vi "PCO_ball_puff_pupil_FLIR_trig_2024_JMR.vi"() -> ()   [LabVIEW 2020]
uses:
  C:/Users/jqr5792/AppData/Roaming/PCO Digital Camera Toolbox/pco.labview/pco.camera/Controls/binning.ctl
  <vilib>/vision/driver/IMAQdx.llb/IMAQdx Camera Control Mode.ctl
  <vilib>/userDefined/High Color/IMAQdx.ctl
  <vilib>/vision/driver/IMAQdx.llb/IMAQdx Acquisition Mode.ctl
  C:/Users/jqr5792/AppData/Roaming/PCO Digital Camera Toolbox/pco.labview/pco.camera/Camera.lvclass
  <vilib>/vision/driver/IMAQdx.llb/IMAQdx Buffer Number Mode.ctl
  7076c1c6-cf5a-4733-8e55-1dfd44238ec2.vi
  <vilib>/DAQmx/write.llb/DAQmx Write (Digital Bool 1Line 1Point).vi
  <vilib>/DAQmx/read.llb/DAQmx Read (Analog 1D Wfm NChan NSamp).vi
  <vilib>/DAQmx/write.llb/DAQmx Write (Digital 1D Bool NChan 1Samp 1Line).vi
  <vilib>/DAQmx/create/channels.llb/DAQmx Create Channel (AI-Voltage-Basic).vi
  <vilib>/DAQmx/configure/timing.llb/DAQmx Timing (Sample Clock).vi
  <vilib>/DAQmx/configure/trigger.llb/DAQmx Start Trigger (Digital Edge).vi
  <vilib>/DAQmx/create/channels.llb/DAQmx Create Channel (DO-Digital Output).vi
  <vilib>/DAQmx/create/channels.llb/DAQmx Create Channel (CO-Pulse Generation-Frequency).vi
  <vilib>/DAQmx/configure/timing.llb/DAQmx Timing (Implicit).vi
  <vilib>/DAQmx/miscellaneous.llb/DAQmx Fill In Error Info.vi
  <vilib>/vision/driver/NI_Vision_Acquisition_Software.lvlib
panel:
  out "New Lost":u32
  out "NewNumLost":u32[](array[numeric])
  out "NewBuffNum":u32[](array[numeric])
  out "Buffer Number Out":u32
  out "Min/Sec for trial":cluster{dbl, dbl}
  in  "No stim":dbl=1.0
  out "n total images":i32
  out "PCO Frame Rate":dbl
  out "Time Elapsed (s)":u32
  out "Recorded Images":u32=7194
  out "PCO Recording":bool=TRUE
  in  "ROI":cluster{"x0":u64, "y0":u64, "x1":u64, "y1":u64}={"x0"=100, "y0"=175, "x1"=500, "y1"=425}
  in  "Binning":T1={"vert"=4, "horz"=4}
  in  "TriggerMode":T2(ring)=enum."external exposure start"
  in  "Exposure [s]":dbl=0.008 min=0.0005 max=2.0 step=0.001
  out "Image":T3(plugin-control)
  out "Last Whisk\nBuffer":u32=488
  out "Actual WhiskCam\nFrame Rate":dbl(knob)=148.05583250249254 scale=0.0..300.0
  out "Pupil":T3(plugin-control)
  out "Solenoids":bool[](array[boolean])
  in  "Stim \nOffset (s)":dbl=15.0
  in  "Puff \nDuration (s)":dbl=0.1 step=0.1
  in  "Inter-Stim\nInterval (s)":dbl=30.0
  in  "Stim only":dbl=5.0
  in  "Auditory control":dbl=2.0
  in  "Left Pad":tag="Dev1/port0/line1"
  in  "Right Pad":tag="Dev1/port0/line3"
  in  "Squeeze":tag="Dev1/port0/line2"
  out "Analog Data":bool
  out "Analog acquisition length":i32
  in  "Channel Labels":string[](array[string])=["BallVelocity", "LeftPad", "Control", "RightPad", "Broadband", "LFP", "MUA"]
  in  "physical channels":tag="Dev1/ai0:6"
  in  "Analog Acquisition Setup":cluster{"Analog Sampling Rate":u16}={"Analog Sampling Rate"=5000} {"Analog Sampling Rate" format="%0.0f"}
  in  "Camera Acquisition Setup":cluster{"CBVCam Rate":u16, "WebCam Rate":u16}={"CBVCam Rate"=60, "WebCam Rate"=30}
  out "Notes Size":i32=7
  out "Notes Reversed":string[](array[string])=["Experimenter", "Animal ID", "Imaged Hemisphere", "Solenoid Pressure", "Isoflurane time", "Session ID", "Amplifier Gain"]
  out "Notes Array":string[](array[string])=["Amplifier Gain", "Session ID", "Isoflurane time", "Solenoid Pressure", "Imaged Hemisphere", "Animal ID", "Experimenter"]
  in  "Session Notes:":T4={"Experimenter"="Joe Ricotta", "Animal ID"="T31", "Imaged Hemisphere"="RH", "Solenoid Pressure"="10", "Infusion Compound"="na", "Infusion volume nL"="na", "Infusion rate nlpS"="na", "Block"="1000", "Molar conc um"="na"}
  in  "Target Path":path=path "D:/Joe/sample/PCO_setup" caption="Final saved file location"
  out "Current file name":string="170828_12_37_58"
  out "Actual WebCam Frame Rate":dbl(knob) scale=0.0..30.0
  out "WebCam":T3(plugin-control)
  out "CBV Camera":bool=TRUE
  out "Trial Time Elapsed (Min)":cluster{dbl, dbl}(slide)={0.5, 0.05364406000000001} scale=0.0..17.0
  in  "Temp Path":path=path "C:/LabView Direct Files" caption="Temporary path for\nstreamed data"
  in  "Stop":bool
  # "File Settings:"
  # "Binning: 4,4"
  # "roi: 50, 200, 600, 400"
  # "Left Pad"
  # "Control"
  # "Right"
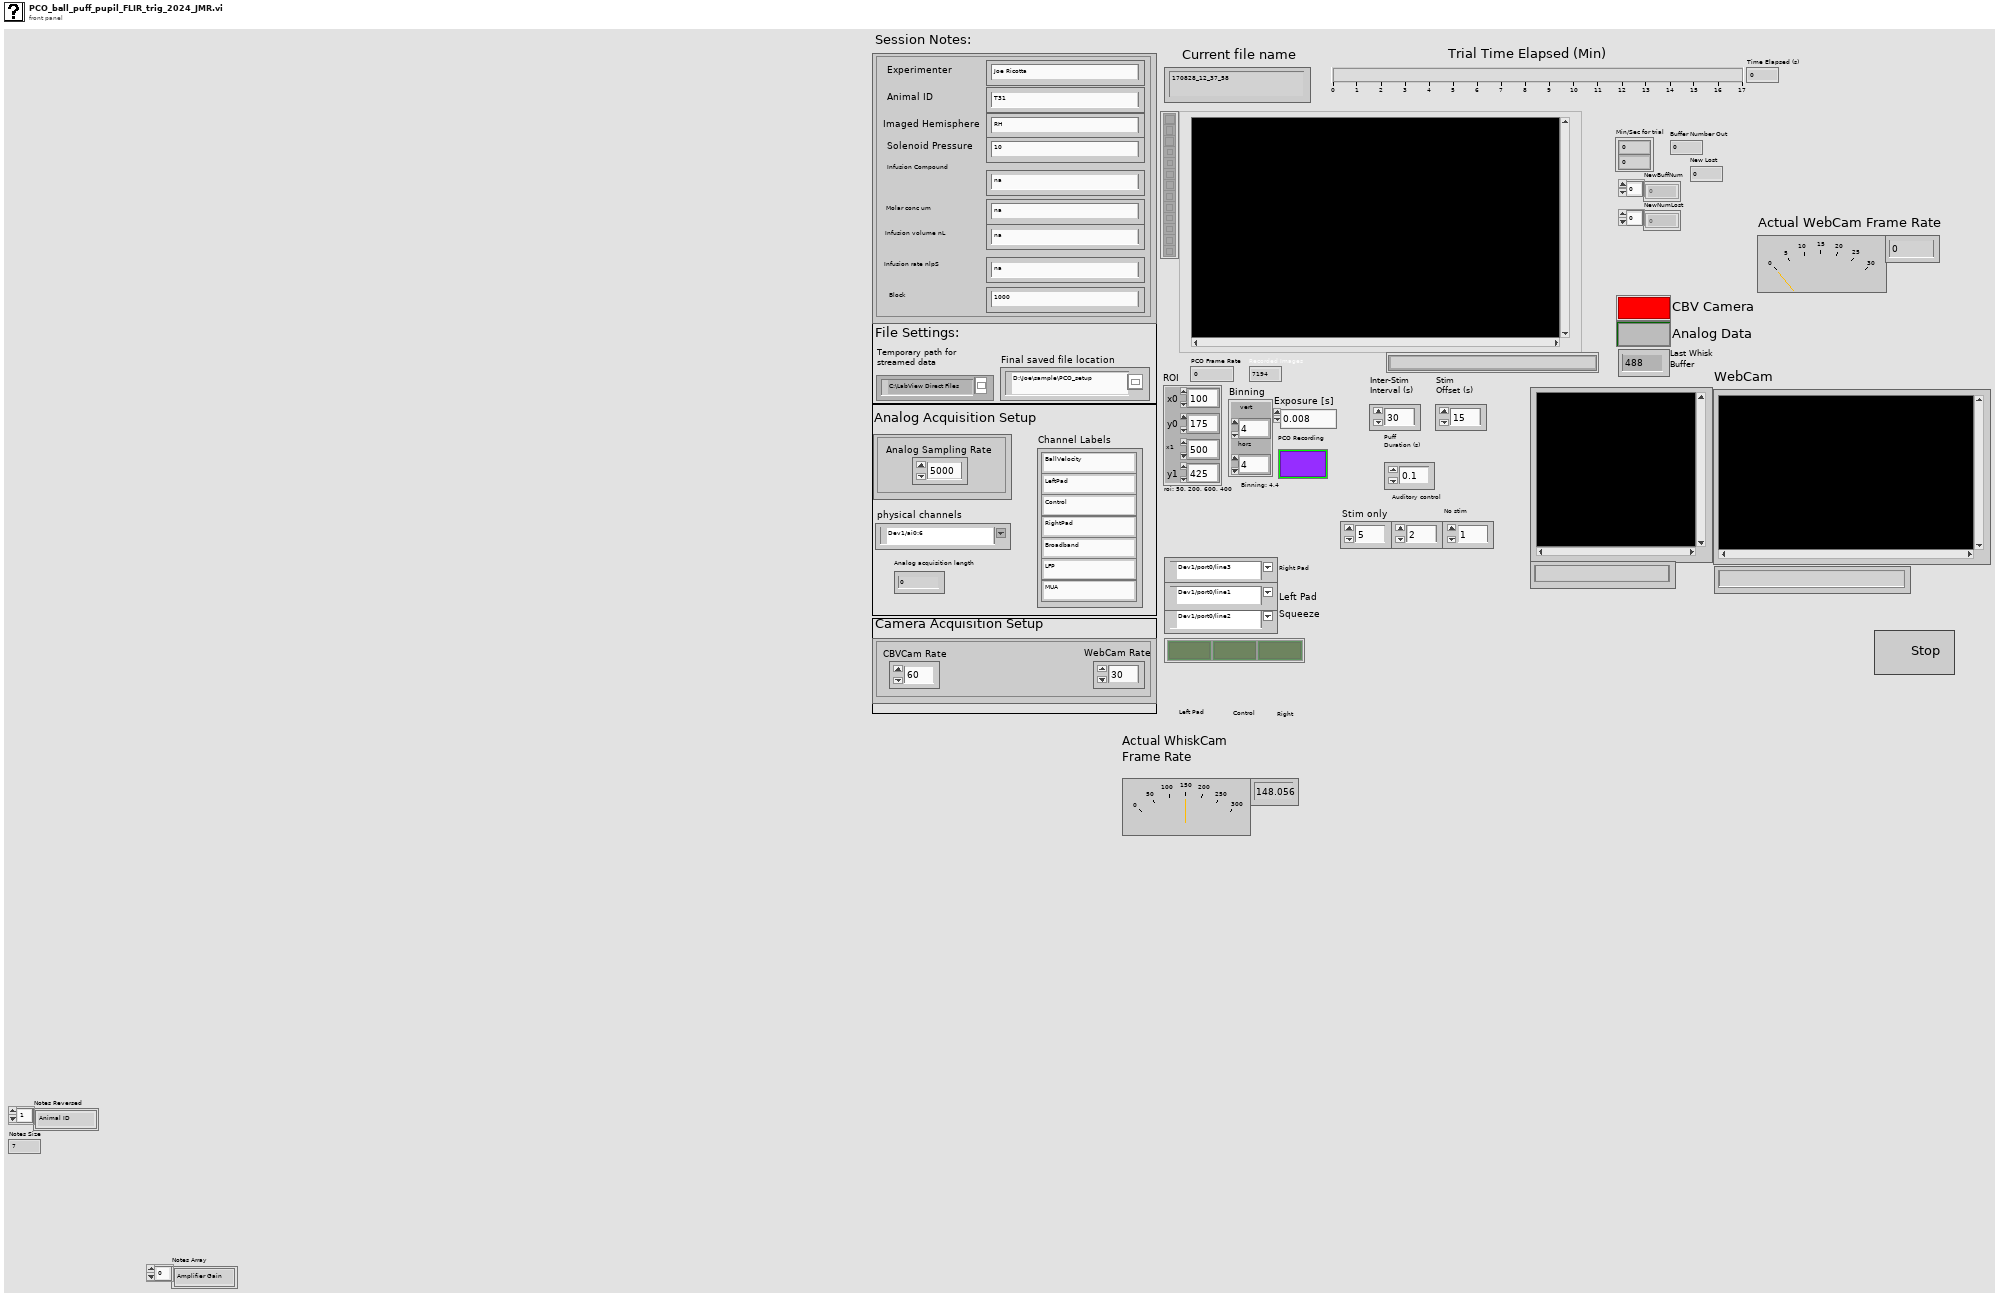
[diagram p1: front panel]
types:
  T1 = typedef "Camera.lvclass/binning.ctl" = cluster{"vert":u16, "horz":u16}
  T2 = enum16{"auto sequence", "software trigger", "external exposure start", "external exposure control"}
  T3 = typedef "IMAQ Image.ctl" = refnum<image>
  T4 = cluster{"Experimenter":string, "Animal ID":string, "Imaged Hemisphere":string, "Solenoid Pressure":string, "Infusion Compound":string, "Infusion volume nL":string, "Infusion rate nlpS":string, "Block":string, "Molar conc um":string}
  T5 = typedef "IMAQdx.ctl" = refnum<k21>
  T6 = typedef "Image Type" = u32
  T7 = enum16{"open", "replace", "create", "open or create", "replace or create", "replace or create with confirmation"}
  T8 = typedef "NI_Vision_Acquisition_Software.lvlib/IMAQdx Acquisition Mode.ctl" = enum32{"One Shot", "Continuous"}
  T9 = typedef "NI_Vision_Acquisition_Software.lvlib/IMAQdx Camera Control Mode.ctl" = enum32{"Controller", "Listener"}
  T10 = enum16{"open", "open or create", "create or replace", "create", "open (read-only)"}
  T11 = cluster{"exposure_time_s":dbl, "delay_time_s":dbl, "roi":cluster{"x0":u64, "y0":u64, "x1":u64, "y1":u64}, "timestamp_mode":u16, "pixelrate":u32, "trigger_mode":u16, "acquire_mode":u16, "metadata_mode":u16, "noisefilter_mode":u16, "binning":T1}
  T12 = typedef "IMAQ AVI2 Refnum.ctl" = refnum<k20>
  T13 = enum16{"sequence", "sequence non blocking", "ring buffer", "fifo", "sequence_dpcore", "sequence_non_blocking_dpcore", "ring_buffer_dpcore", "fifo_dpcore", "tif", "multitif", "pcoraw", "b16", "dicom", "multidicom"}
  T14 = enum16{"Undefined", "Mono8", "Mono16", "BGRA8", "RGBA8", "BGRA16", "RGBA16", "CompressedMono8"}
  T15 = enum16{"big-endian, network order", "native, host order", "little-endian"}
  T16 = typedef "NI_Vision_Acquisition_Software.lvlib/IMAQdx Buffer Number Mode.ctl" = enum32{"Next", "Last", "Buffer Number", "Every", "Last New"}
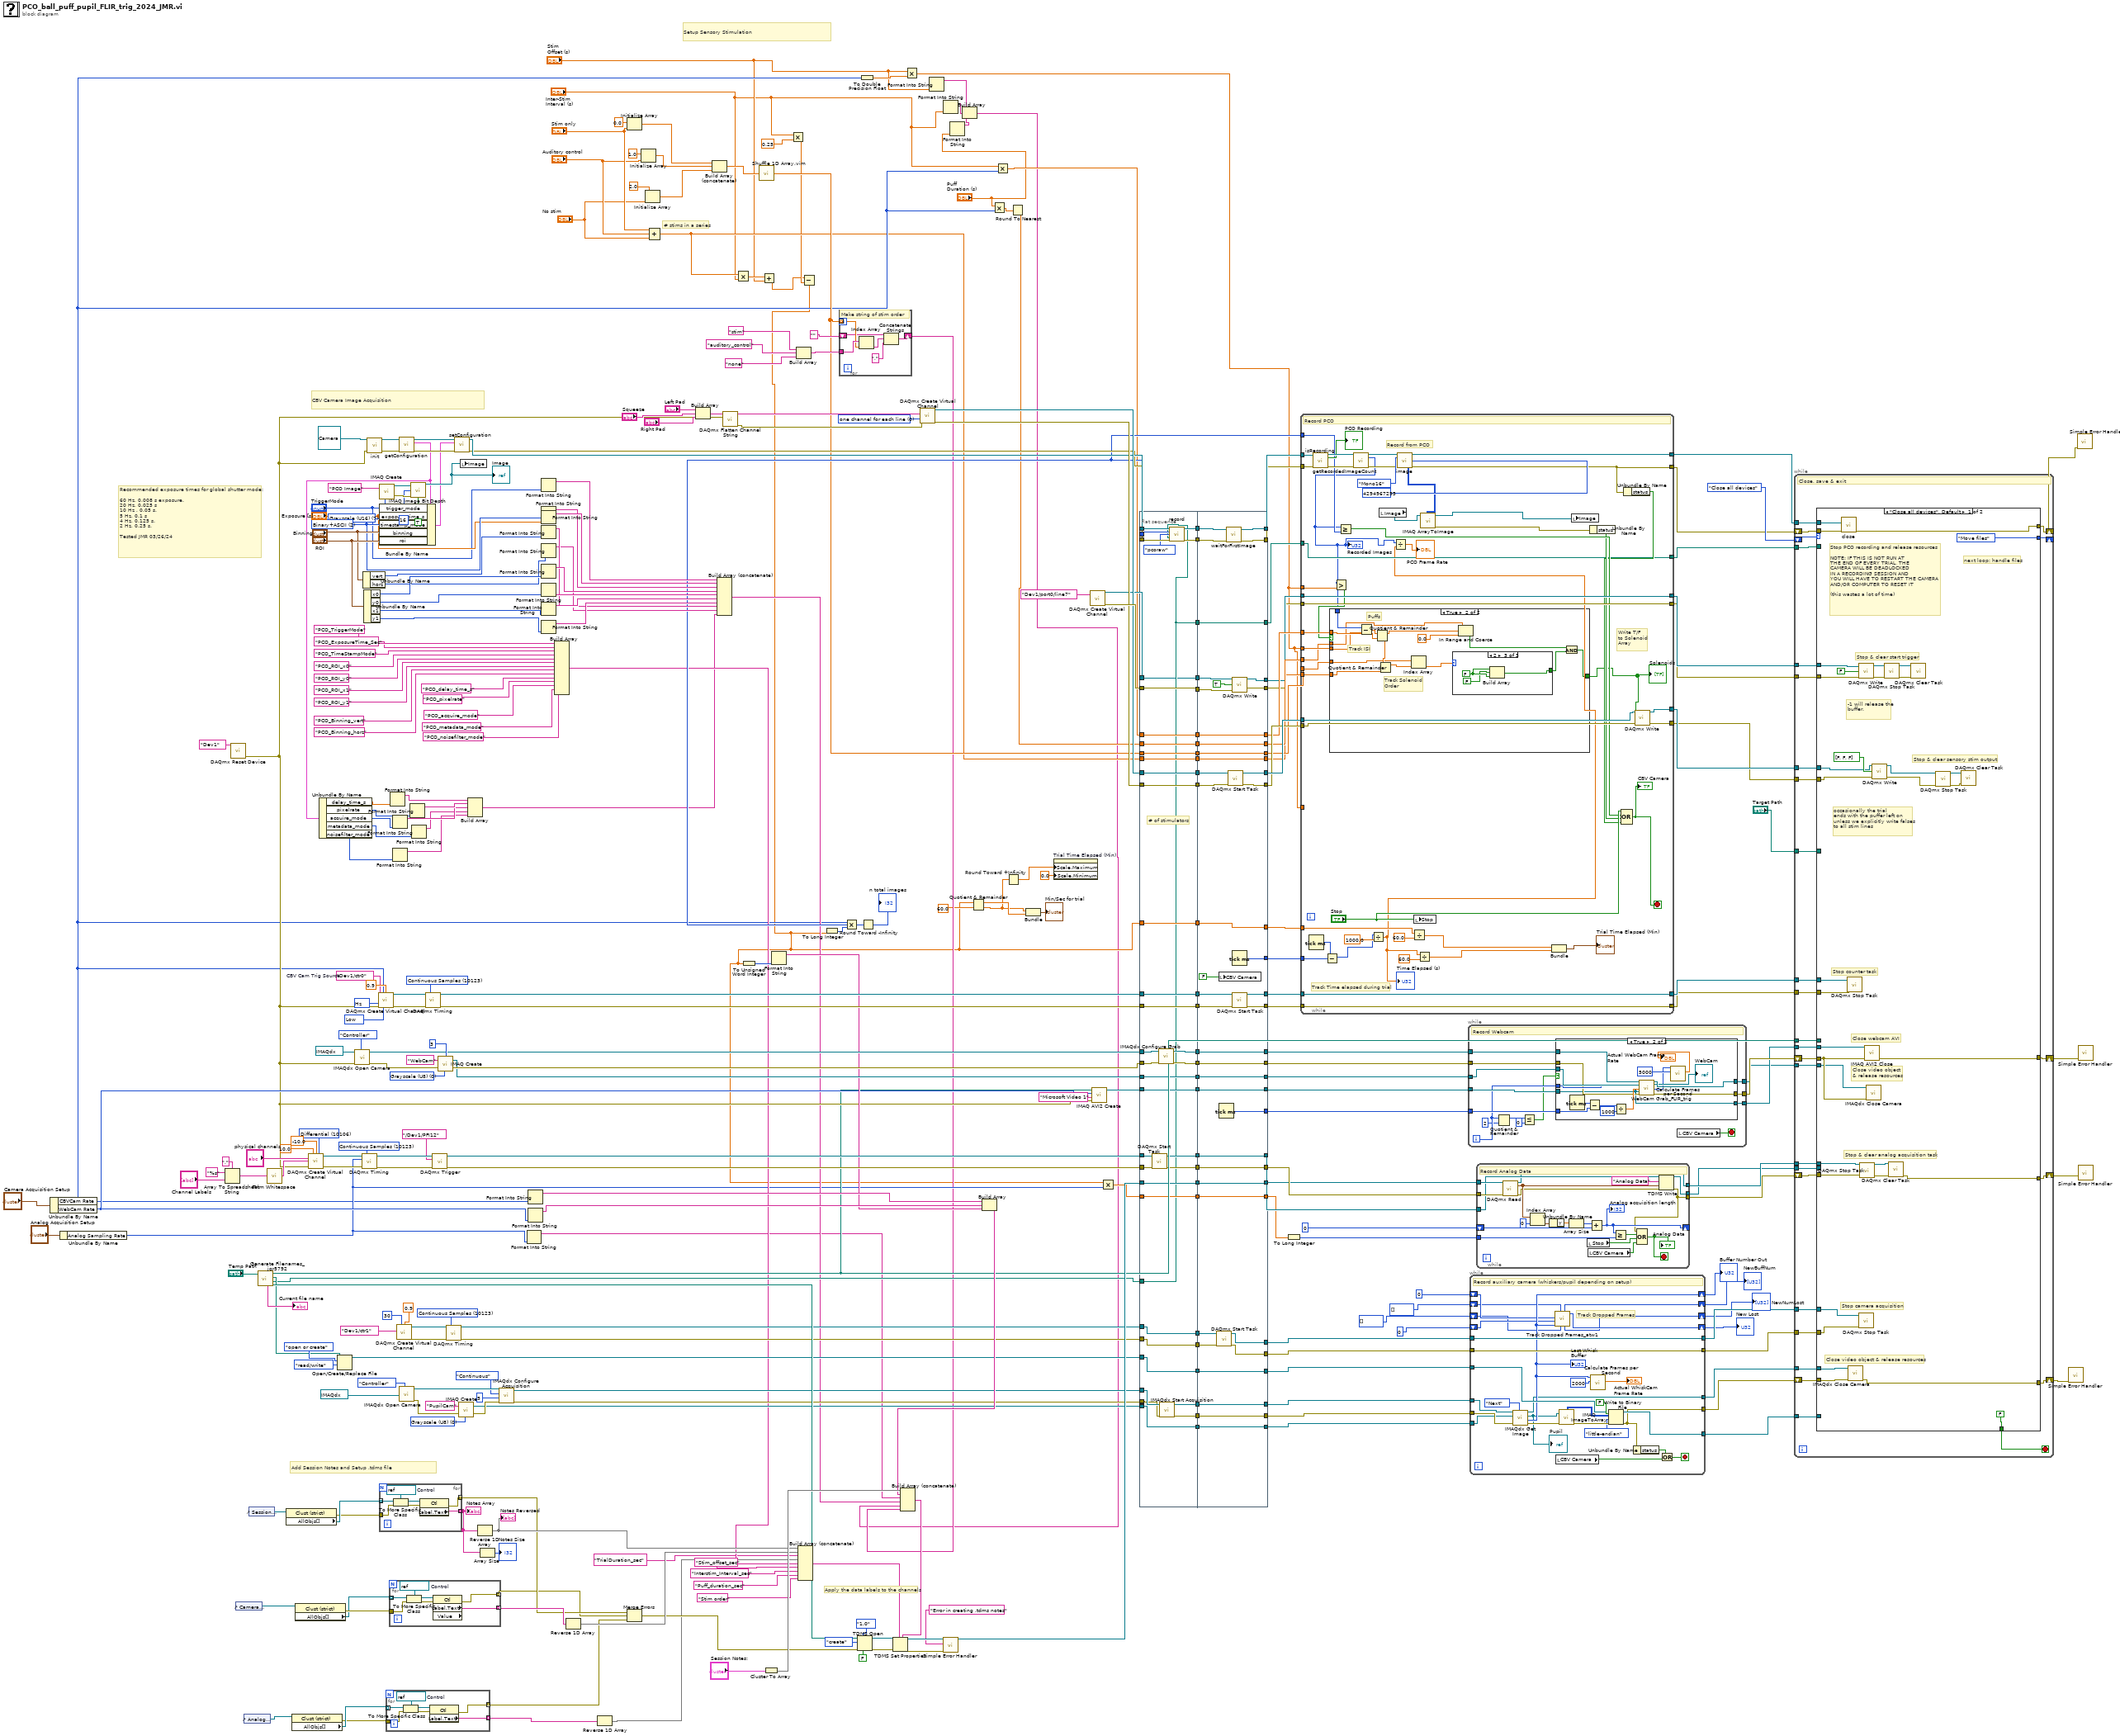
[diagram p0: block diagram]
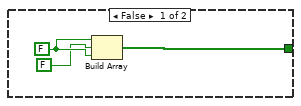
[diagram p2: hidden frame]
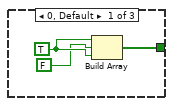
[diagram p3: hidden frame]
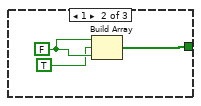
[diagram p4: hidden frame]
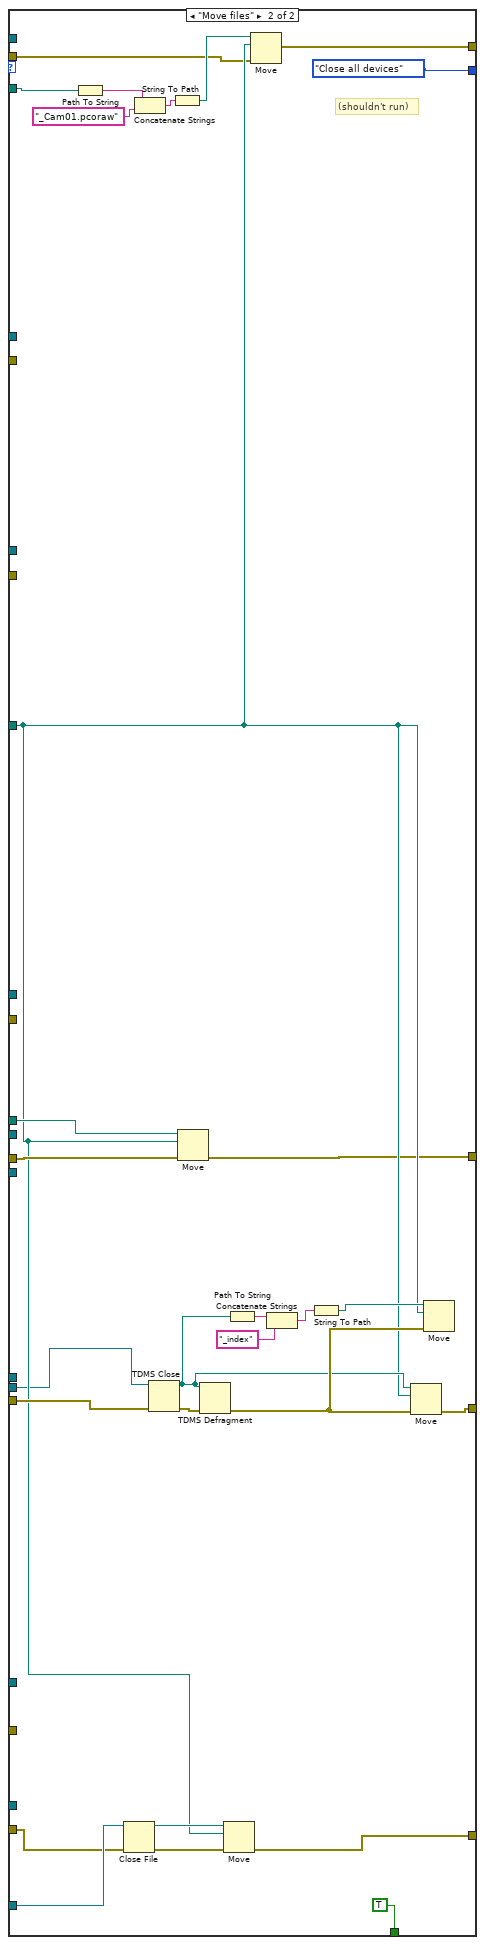
[diagram p5: hidden frame]
diagram:
  w118 = u16 2 items=["OFF", "Binary", "Binary+ASCII", "ASCII"] ("wTimeStampMode")
  w149 = T6 7 items=["Grayscale (U8)", "Grayscale (I16)", "Grayscale (SGL)", "Complex (CSG)", "RGB (U32)", "HSL (U32)", "RGB (U64)", "Grayscale (U16)"] ("Image Type")
  w179 = 10123 items=["Finite Samples"=10178, "Continuous Samples"=10123, "Hardware Timed Single Point"=12522] ("sample mode")
  w184 = T6 0 items=["Grayscale (U8)", "Grayscale (I16)", "Grayscale (SGL)", "Complex (CSG)", "RGB (U32)", "HSL (U32)", "RGB (U64)", "Grayscale (U16)"] ("Image Type")
  w222 = 0 items=["one channel for each line", "one channel for all lines"] ("line grouping")
  w225 = tag "Dev1/ctr0"  # CBV Cam Trig Source
  w298 = 10123 items=["Finite Samples"=10178, "Continuous Samples"=10123, "Hardware Timed Single Point"=12522] ("sample mode")
  w301 = 10106 items=["default"=-1, "RSE"=10083, "NRSE"=10078, "Differential"=10106, "Pseudodifferential"=12529] ("input terminal configuration")
  w321 = T6 0 items=["Grayscale (U8)", "Grayscale (I16)", "Grayscale (SGL)", "Complex (CSG)", "RGB (U32)", "HSL (U32)", "RGB (U64)", "Grayscale (U16)"] ("Image Type")
  w326 = 10123 items=["Finite Samples"=10178, "Continuous Samples"=10123, "Hardware Timed Single Point"=12522] ("sample mode")
  w329 = 10373 items=["Hz"=10373] ("units")
  w330 = 10214 items=["High"=10192, "Low"=10214] ("idle state")
  # "Recommended exposure times for global shutter mode:\n\n60 Hz, 0.008 s exposure.\n20 Hz, 0.025 s\n10 Hz , 0.05 s.\n5 Hz, 0.1 s\n4 Hz, 0.125 s.\n2 Hz, 0.25 s.\n\nTested JMR 03/26/24"
  # "Setup Sensory Stimulation"
  # "# stims in a series"
  # "Apply the data labels to the channels"
  # "CBV Camera Image Acquisition"
  # "Add Session Notes and Setup .tdms file"
  n1 = Unbundle By Name "Unbundle By Name"("Camera Acquisition Setup") -> ("CBVCam Rate"=w26:u16, "WebCam Rate"=w155:u16)
  n2 = Unbundle By Name("Analog Acquisition Setup") -> ("Analog Sampling Rate"=w65:u16)
  n3 = Array To Spreadsheet String(delimiter (Tab)=",", array="Channel Labels", 3:"%s" ("format string")) -> (spreadsheet string=w239:string)
  n4 = call <vilib>:"DAQmx Reset Device.vi"("device in"=tag "Dev1") -> ("error out"=w101:errorcluster)  [unwired: 14 in]
  n5 = control-ref of="Camera Acquisition Setup"() -> (w252:refnum<vi>)
  n6 = control-ref of="Analog Acquisition Setup"() -> (w251:refnum<vi>)
  n7 = control-ref of="Session Notes:"() -> (w275:refnum<vi>)
  n8 = call "Generate Filenames_jqr5792.vi"("path"="Temp Path") -> ("TDMS Path"=w269:path, "PCO Path"=w111:path, "Basler Path"=w176:path, "WebCam Path"=w79:path, "Analog file name"=→"Current file name":string)  [unwired: 5 in, 1 out]
  n9 = call <vilib>:"Trim Whitespace.vi"("string"=w239) -> ("trimmed string"=w238:string)  [unwired: 1 in]
  n10 = property class="Clust (strict)"(reference=w275) -> (error out=w278:errorcluster, "AllObjs[]"=w279:refnum<vi>[])  [unwired: 1 in, 1 out]
  n11 = property class="Clust (strict)"(reference=w251) -> (error out=w249:errorcluster, "AllObjs[]"=w250:refnum<vi>[])  [unwired: 1 in, 1 out]
  n12 = property class="Clust (strict)"(reference=w252) -> (error out=w273:errorcluster, "AllObjs[]"=w272:refnum<vi>[])  [unwired: 1 in, 1 out]
  n13 = call-poly <vilib>:"DAQmx Create Virtual Channel.vi"("maximum value"=10.0, "minimum value"=-10.0, "input terminal configuration"=w301, "physical channels"="physical channels", "name to assign"=w238, "error in"=w101) -> ("task out"=w300:refnum<k21>, "error out"=w299:errorcluster)  [unwired: 8 in]
  n14 = Open/Create/Replace File(file path (use dialog)=w176, operation (0:open)=T7."open or create", access (0:read/write)=enum16{"read/write", "read-only", "write-only"}."read/write") -> (refnum out=w160:refnum<file>)  [unwired: 3 in, 2 out]
  n15 = call <vilib>:"IMAQdx Open Camera.vi"("Camera Control Mode"=IMAQdx_Camera_Control_Mode."Controller", "error in"=w101, "Session In"=T5 "cam9") -> ("error out"=w318:errorcluster, "Session Out"=w316:T5)  [unwired: 7 in]
  n16 = call-poly <vilib>:"DAQmx Timing.vi"("task/channels in"=w300, "sample mode"=w298, "rate"=w65, "error in"=w299) -> ("task out"=w297:refnum<k21>, "error out"=w296:errorcluster)  [unwired: 10 in]
  n17 = Unbundle By Name("Binning") -> ("vert"=w119:u16, "horz"=w120:u16)
  n18 = Unbundle By Name("ROI") -> ("x0"=w121:u64, "y0"=w122:u64, "x1"=w123:u64, "y1"=w124:u64)
  n19 = call-dynamic "init.vi"("Camera in"=refnum<class "Camera.lvclass"> refnum ("PCOCamera in"), "error in (no error)"=w101) -> ("Camera out"=w146:refnum<class "Camera.lvclass">, "error out"=w145:errorcluster)  [unwired: 7 in]
  n20 = call-poly <vilib>:"DAQmx Create Virtual Channel.vi"("frequency"=w26, "duty cycle"=0.9, "counter"=w225, "units"=w329, "error in"=w101, "idle state"=w330) -> ("task out"=w328:refnum<k21>, "error out"=w327:errorcluster)  [unwired: 8 in]
  n21 = call "IMAQ Create"("Image Name"="PCO Image", "Image Type"=w149) -> ("New Image"=w39:T3, "error out"=w148:errorcluster)  [unwired: 3 in]
  n22 = for {
    tunnel: [w335] -> w277 mode=indexing
    tunnel: w279 -> [w334] mode=indexing
    tunnel: w278 -> [w333]
    tunnel: [w331] -> w258 mode=indexing
    w336 = refnum<vi> refnum  # Control
    n23 = To More Specific Class(target class=w336, reference=w334, error in=w333) -> (specific class reference=w337:refnum<vi>, error out=w332:errorcluster)
    n24 = property class="Ctl"(reference=w337, error in=w332) -> (error out=w331:errorcluster, "Label.Text"=w335:string)  [unwired: 1 out]
  }
  "Notes Array" <- w277
  n25 = for {
    tunnel: [w342] -> w247 mode=indexing
    tunnel: w250 -> [w341] mode=indexing
    tunnel: w249 -> [w340]
    tunnel: [w338] -> w248 mode=indexing
    w343 = refnum<vi> refnum  # Control
    n26 = To More Specific Class(target class=w343, reference=w341, error in=w340) -> (specific class reference=w344:refnum<vi>, error out=w339:errorcluster)
    n27 = property class="Ctl"(reference=w344, error in=w339) -> (error out=w338:errorcluster, "Label.Text"=w342:string)  [unwired: 1 out]
  }
  n28 = for {
    tunnel: [w349] -> w274 mode=indexing
    tunnel: w272 -> [w348] mode=indexing
    tunnel: w273 -> [w347]
    tunnel: [w345] -> w257 mode=indexing
    w350 = refnum<vi> refnum  # Control
    n29 = To More Specific Class(target class=w350, reference=w348, error in=w347) -> (specific class reference=w351:refnum<vi>, error out=w346:errorcluster)
    n30 = property class="Ctl" props=["Label", "Text", "Value"](reference=w351, error in=w346) -> (error out=w345:errorcluster, "Label.Text"=w349:string)  [unwired: 2 out]
  }
  n31 = call-poly <vilib>:"DAQmx Create Virtual Channel.vi"("frequency"=30, "duty cycle"=0.9, "counter"=tag "Dev1/ctr1" ("Whisker Cam\nTrigger Source")) -> ("task out"=w181:refnum<k21>, "error out"=w180:errorcluster)  [unwired: 11 in]
  n32 = call-dynamic "getConfiguration.vi"("error in (no error)"=w145, "Camera in"=w146) -> ("error out"=w144:errorcluster, "configuration"=w63:T11, "Camera out"=w147:refnum<class "Camera.lvclass">)  [unwired: 7 in]
  n33 = Unbundle By Name(w63) -> ("delay_time_s"=w57:dbl, "pixelrate"=w56:u32, "acquire_mode"=w55:u16, "metadata_mode"=w54:u16, "noisefilter_mode"=w53:u16)
  n34 = Bundle By Name(cluster=w63, "trigger_mode"="TriggerMode", "exposure_time_s"="Exposure [s]", "timestamp_mode"=w118, "binning"="Binning", "roi"="ROI") -> (w143:T11)
  n35 = Format Into String(w57) -> (resulting string=w52:string)  [unwired: 3 in, 1 out]
  n36 = Format Into String(w53) -> (resulting string=w48:string)  [unwired: 3 in, 1 out]
  n37 = Format Into String(w55) -> (resulting string=w50:string)  [unwired: 3 in, 1 out]
  n38 = call <vilib>:"IMAQdx Open Camera.vi"("Camera Control Mode"=IMAQdx_Camera_Control_Mode."Controller", "Session In"=T5 "cam5" ("Pupil Cam")) -> ("error out"=w187:errorcluster, "Session Out"=w190:T5)  [unwired: 8 in]
  n39 = Format Into String(w56) -> (resulting string=w51:string)  [unwired: 3 in, 1 out]
  n40 = call "IMAQ Image Bit Depth"("Image"=w39, "Bit Depth (0)"=u32 16, "error in (no error)"=w148, "Get/Set Bit Depth? (Set)"=TRUE) -> ("Image Out"=w150:T3)  [unwired: 9 in, 2 out]
  "Image" <- w150
  n41 = Format Into String(w54) -> (resulting string=w49:string)  [unwired: 3 in, 1 out]
  n42 = call-poly <vilib>:"DAQmx Timing.vi"("task/channels in"=w328, "sample mode"=w326, "error in"=w327) -> ("task out"=w285:refnum<k21>, "error out"=w283:errorcluster)  [unwired: 11 in]
  n43 = call-poly <vilib>:"DAQmx Trigger.vi"("task/channels in"=w297, "source"=tag "/Dev1/PFI12", "error in"=w296) -> ("task out"=w294:refnum<k21>, "error out"=w293:errorcluster)  [unwired: 11 in]
  n44 = call "IMAQ Create"("Border Size"=3, "Image Name"="WebCam", "Image Type"=w321, "error in (no error)"=w318) -> ("New Image"=w315:T3, "error out"=w317:errorcluster)  [unwired: 1 in]
  n45 = call-poly <vilib>:"DAQmx Timing.vi"("task/channels in"=w181, "sample mode"=w179, "error in"=w180) -> ("task out"=w169:refnum<k21>, "error out"=w167:errorcluster)  [unwired: 11 in]
  n46 = call-dynamic "setConfiguration.vi"("error in (no error)"=w144, "configuration"=w143, "Camera in"=w147) -> ("error out"=w112:errorcluster, "Camera out"=w113:refnum<class "Camera.lvclass">)  [unwired: 7 in]
  n47 = call "IMAQ Create"("Image Name"="PupilCam", "Image Type"=w184, "error in (no error)"=w187) -> ("New Image"=w163:T3, "error out"=w185:errorcluster)  [unwired: 2 in]
  n48 = local write "Image"(w150) -> ()
  n49 = Build Array(w52, w51, w50, w49, w48) -> (w47:string[])
  n50 = Reverse 1D Array(array=w277) -> (reversed array=w263:string[])
  "Notes Reversed" <- w263
  n51 = Array Size(array=w277) -> (size(s)=→"Notes Size":i32)
  n52 = call <vilib>:"IMAQdx Configure Acquisition.vi"("error in"=w185, "Number of Buffers"=u32 5, "Continuous?"=IMAQdx_Acquisition_Mode."Continuous", "Session In"=w190) -> ("error out"=w164:errorcluster, "Session Out"=w165:T5)  [unwired: 6 in]
  n53 = Format Into String(w65) -> (resulting string=w64:string)  [unwired: 3 in, 1 out]
  n54 = Format Into String(w26) -> (resulting string=w245:string)  [unwired: 3 in, 1 out]
  n55 = Format Into String(w155) -> (resulting string=w244:string)  [unwired: 3 in, 1 out]
  n56 = Format Into String("TriggerMode") -> (resulting string=w131:string)  [unwired: 3 in, 1 out]
  n57 = Format Into String(w118) -> (resulting string=w129:string)  [unwired: 3 in, 1 out]
  n58 = Format Into String("Exposure [s]") -> (resulting string=w130:string)  [unwired: 3 in, 1 out]
  n59 = Format Into String(w119) -> (resulting string=w115:string)  [unwired: 3 in, 1 out]
  n60 = Format Into String(w120) -> (resulting string=w114:string)  [unwired: 3 in, 1 out]
  n61 = Format Into String(w121) -> (resulting string=w128:string)  [unwired: 3 in, 1 out]
  n62 = Format Into String(w122) -> (resulting string=w127:string)  [unwired: 3 in, 1 out]
  n63 = Format Into String(w123) -> (resulting string=w126:string)  [unwired: 3 in, 1 out]
  n64 = Format Into String(w124) -> (resulting string=w125:string)  [unwired: 3 in, 1 out]
  n65 = Build Array("PCO_TriggerMode", "PCO_ExposureTime_Sec", "PCO_TimeStampMode", "PCO_ROI_x0", "PCO_ROI_y0", "PCO_ROI_x1", "PCO_ROI_y1", "PCO_Binning_vert", "PCO_Binning_horz", "PCO_delay_time_s", "PCO_pixelrate", "PCO_acquire_mode", "PCO_metadata_mode", "PCO_noisefilter_mode") -> (w69:string[])
  n66 = Reverse 1D Array(array=w274) -> (reversed array=w262:string[])
  n67 = Reverse 1D Array(array=w247) -> (reversed array=w246:string[])
  n68 = Initialize Array(0.0 ("element"), "Stim only") -> (w219:dbl[])
  n69 = Merge Errors(w258, w257, w248) -> (w256:errorcluster)
  n70 = Initialize Array(1.0 ("element"), "Auditory control") -> (w218:dbl[])
  n71 = Initialize Array(2.0 ("element"), "No stim") -> (w34:dbl[])
  n72 = Compound Arithmetic op=ADD("Stim only", "Auditory control", "No stim") -> (w24:dbl)
  n73 = Build Array("Left Pad", "Squeeze", "Right Pad") -> (w223:tag[])
  n74 = Build Array (concatenate)(w219, w218, w34) -> (w40:dbl[])
  n75 = Build Array (concatenate)(w131, w130, w129, w128, w127, w126, w125, w115, w114, w47) -> (w68:string[])
  n76 = call <vilib>:"DAQmx Flatten Channel String.vi"("names in"=w223, "error in"=w101) -> ("names out"=w198:string, "error out"=w199:errorcluster)  [unwired: 12 in]
  n77 = Multiply(x=w24, y="Inter-Stim\nInterval (s)") -> (x*y=w23:dbl)
  n78 = call "Shuffle 1D Array.vim"("array"=w40) -> ("shuffled array"=w28:dbl[])  [unwired: 4 in]
  n79 = Add(x=w23, y="Stim \nOffset (s)") -> (x+y=w14:dbl)
  n80 = Cluster To Array(cluster="Session Notes:") -> (array=w270:string[])
  n81 = Multiply(x="Inter-Stim\nInterval (s)", y=0.25) -> (x*y=w15:dbl)
  n82 = Build Array("stim", "auditory_control", "none") -> (w30:string[])
  n83 = Build Array (concatenate)(w263, w262, "TrialDuration_sec", w246, w69, "Stim_offset_sec" ("array"), "Interstim_Interval_sec" ("array"), "Puff_duration_sec" ("array"), "Stim order" ("array")) -> (w260:string[])
  n84 = Subtract(x=w14, y=w15) -> (x-y=w13:dbl)
  n85 = To Unsigned Word Integer(number=w13) -> (unsigned 16bit integer=w235:u16)
  n86 = Format Into String(w235) -> (resulting string=w236:string)  [unwired: 3 in, 1 out]
  n87 = To Long Integer(number=w13) -> (32bit integer=w106:i32)
  n88 = for {
    tunnel: w30 -> [w357]
    shift-right: [w354] -> w27
    shift-left: "" -> [w353]
    tunnel: w28 -> [w356] mode=indexing
    # "Make string of stim order"
    n89 = Index Array(array=w357, index=w356) -> (element=w355:string)
    n90 = Concatenate Strings(w353, w355, "," ("string")) -> (w354:string)
  }
  n91 = Multiply(x=w26, y=w106) -> (x*y=w105:i32)
  n92 = TDMS Open(6:FALSE ("disable buffering? (T)"), 7:enum16{"1.0", "2.0"}."1.0" ("file format version (2.0)"), 8:w256, 10:T10."create" ("operation (0:open)"), 11:w269) -> (0:w264:errorcluster, 3:w265:refnum<k34>)  [unwired: 2 in]
  n93 = To Double Precision Float(number=w26) -> (double precision float=w216:dbl)
  n94 = Round Toward -Infinity(1:w105) -> (0:w104:i32)
  "n total images" <- w104
  n95 = Multiply(x="Stim \nOffset (s)", y=w216) -> (x*y=w11:dbl)
  n96 = call-poly <vilib>:"DAQmx Create Virtual Channel.vi"("lines"=w198, "line grouping"=w222, "error in"=w199) -> ("task out"=w214:refnum<k21>, "error out"=w212:errorcluster)  [unwired: 11 in]
  n97 = Format Into String("Stim \nOffset (s)") -> (resulting string=w43:string)  [unwired: 3 in, 1 out]
  n98 = Format Into String("Inter-Stim\nInterval (s)") -> (resulting string=w42:string)  [unwired: 3 in, 1 out]
  n99 = Format Into String("Puff \nDuration (s)") -> (resulting string=w41:string)  [unwired: 3 in, 1 out]
  n100 = Build Array(w43, w42, w41) -> (w1:string[])
  n101 = Quotient & Remainder(x=w13, y=60.0) -> (x-y*floor(x/y)=w22:dbl, floor(x/y)=w19:dbl)
  n102 = Build Array(w245, w244, w236) -> (w243:string[])
  n103 = Build Array (concatenate)(w270, w243, w64, w68, w1, w27) -> (w261:string[])
  n104 = TDMS Set Properties(5:w261, 7:w260, 8:w264, 11:w265) -> (0:w255:errorcluster, 3:w259:refnum<k34>)  [unwired: 2 in, 2 out]
  n105 = call <vilib>:"Simple Error Handler.vi"("error source (\" \")"="Error in creating .tdms notes" ("error source (\" \")"), "error in (no error)"=w255) -> ()  [unwired: 3 in, 5 out]
  n106 = Multiply(x="Puff \nDuration (s)", y=w26) -> (x*y=w217:dbl)
  n107 = Multiply(x="Inter-Stim\nInterval (s)", y=w26) -> (x*y=w9:dbl)
  n108 = Round Toward +Infinity(x=w19) -> (ceil(x): smallest int >= x=w18:dbl)
  n109 = Round To Nearest(number=w217) -> (nearest integer value=w7:dbl)
  n110 = Bundle(w19, w22) -> (→"Min/Sec for trial":cluster{dbl, dbl})  [unwired: 1 in]
  n111 = property on="Trial Time Elapsed (Min)" class="Slide (strict)"("Scale.Maximum"=w18, "Scale.Minimum"=0.0 ("Scale.Range:Minimum")) -> ()  [unwired: 2 in, 2 out]
  n112 = call-poly <vilib>:"DAQmx Create Virtual Channel.vi"("lines"=tag "Dev1/port0/line7") -> ("task out"=w98:refnum<k21>, "error out"=w228:errorcluster)  [unwired: 13 in]
  n113 = call "IMAQ AVI2 Create"("error in (no error)"=w101, "Codec"="Microsoft Video 1", "Frames Per Second"=w155, "AVI Path"=w79) -> ("AVI Refnum"=w154:T12)  [unwired: 6 in, 1 out]
  n114 = Multiply(x=w13, y=w65) -> (x*y=w233:dbl)
  n115 = flat-sequence {
    tunnel: w317 -> [w395]
    tunnel: w316 -> [w394]
    tunnel: w315 -> [w393]
    tunnel: [w393] -> w314
    tunnel: [w392] -> w312
    tunnel: [w391] -> w310
    tunnel: w154 -> [w390]
    tunnel: [w390] -> w308
    tunnel: w13 -> [w389]
    tunnel: [w389] -> w302
    tunnel: w294 -> [w388]
    tunnel: w293 -> [w387]
    tunnel: [w386] -> w292
    tunnel: [w385] -> w291
    tunnel: [w384] -> w286
    tunnel: w259 -> [w384]
    tunnel: w285 -> [w383]
    tunnel: [w383] -> w284
    tunnel: w283 -> [w382]
    tunnel: [w382] -> w282
    tunnel: w233 -> [w381]
    tunnel: [w381] -> w232
    tunnel: w228 -> [w380]
    tunnel: [w380] -> w227
    tunnel: w214 -> [w379]
    tunnel: [w379] -> w213
    tunnel: w212 -> [w378]
    tunnel: [w378] -> w211
    tunnel: [w377] -> w207
    tunnel: w9 -> [w377]
    tunnel: w7 -> [w376]
    tunnel: [w376] -> w206
    tunnel: w28 -> [w375]
    tunnel: [w375] -> w204
    tunnel: w24 -> [w374]
    tunnel: [w374] -> w202
    tunnel: [w373] -> w173
    tunnel: [w372] -> w171
    tunnel: w169 -> [w371]
    tunnel: [w371] -> w168
    tunnel: w167 -> [w370]
    tunnel: [w370] -> w166
    tunnel: w165 -> [w369]
    tunnel: [w368] -> _
    tunnel: w164 -> [w368]
    tunnel: w163 -> [w367]
    tunnel: [w367] -> w162
    tunnel: w160 -> [w366]
    tunnel: [w366] -> w159
    tunnel: w113 -> [w365]
    tunnel: w112 -> [w364]
    tunnel: w111 -> [w359]
    tunnel: [w362] -> w110
    tunnel: [w361] -> w109
    tunnel: w104 -> [w360]
    tunnel: [w359] -> w103
    tunnel: w98 -> [w358]
    tunnel: [w358] -> w97
    tunnel: [w437] -> w319
    tunnel: w314 -> [w436]
    tunnel: [w436] -> w313
    tunnel: w312 -> [w435]
    tunnel: [w435] -> w311
    tunnel: w310 -> [w434]
    tunnel: [w434] -> w309
    tunnel: w308 -> [w433]
    tunnel: [w433] -> w307
    tunnel: [w427] -> w306
    tunnel: [w426] -> w305
    tunnel: [w432] -> w304
    tunnel: [w431] -> w303
    tunnel: w302 -> [w431]
    tunnel: [w430] -> w289
    tunnel: w292 -> [w430]
    tunnel: [w429] -> w290
    tunnel: w291 -> [w429]
    tunnel: [w428] -> w287
    tunnel: w286 -> [w428]
    tunnel: w284 -> [w425]
    tunnel: w282 -> [w424]
    tunnel: w232 -> [w423]
    tunnel: [w423] -> w231
    tunnel: w227 -> [w400]
    tunnel: w213 -> [w421]
    tunnel: w211 -> [w420]
    tunnel: [w419] -> w210
    tunnel: [w418] -> w209
    tunnel: [w417] -> w208
    tunnel: w207 -> [w417]
    tunnel: w206 -> [w416]
    tunnel: [w416] -> w205
    tunnel: w204 -> [w415]
    tunnel: [w415] -> w203
    tunnel: w202 -> [w414]
    tunnel: [w414] -> w201
    tunnel: [w413] -> w175
    tunnel: [w412] -> w174
    tunnel: w173 -> [w411]
    tunnel: [w411] -> w172
    tunnel: w171 -> [w410]
    tunnel: [w410] -> w170
    tunnel: w168 -> [w409]
    tunnel: w166 -> [w408]
    tunnel: w162 -> [w407]
    tunnel: [w407] -> w161
    tunnel: w159 -> [w406]
    tunnel: [w406] -> w158
    tunnel: w110 -> [w405]
    tunnel: w109 -> [w404]
    tunnel: [w403] -> w108
    tunnel: [w402] -> w107
    tunnel: [w401] -> w102
    tunnel: w103 -> [w401]
    tunnel: [w399] -> w100
    tunnel: [w398] -> w99
    tunnel: w97 -> [w396]
    frame #0 {
      # "# of stimulators"
      n116 = call <vilib>:"DAQmx Start Task.vi"("task/channels in"=w388, "error in"=w387) -> ("task out"=w386:refnum<k21>, "error out"=w385:errorcluster)  [unwired: 12 in]
      n117 = call <vilib>:"IMAQdx Configure Grab.vi"("error in"=w395, "Session In"=w394) -> ("error out"=w391:errorcluster, "Session Out"=w392:T5)  [unwired: 8 in]
      n118 = call <vilib>:"IMAQdx Start Acquisition.vi"("error in"=w368, "Session In"=w369) -> ("error out"=w372:errorcluster, "Session Out"=w373:T5)  [unwired: 8 in]
      n119 = call-dynamic "record.vi"("Camera in"=w365, "num_images"=w360, "record_mode"=T13."pcoraw", "file_path"=w359, "error in (no error)"=w364) -> ("Camera out"=w362:refnum<class "Camera.lvclass">, "error out"=w361:errorcluster)  [unwired: 9 in]
    }
    frame #1 {
      n120 = call <vilib>:"DAQmx Start Task.vi"("task/channels in"=w409, "error in"=w408) -> ("task out"=w413:refnum<k21>, "error out"=w412:errorcluster)  [unwired: 12 in]
      n121 = local write "CBV Camera"(FALSE ("Finished Acquiring")) -> ()
      n122 = Tick Count (ms)() -> (millisecond timer value=w437:u32)
      n123 = call-dynamic "waitForFirstImage.vi"("error in (no error)"=w404, "Camera in"=w405) -> ("error out"=w402:errorcluster, "Camera out"=w403:refnum<class "Camera.lvclass">)  [unwired: 8 in]
      n124 = call <vilib>:"DAQmx Start Task.vi"("task/channels in"=w421, "error in"=w420) -> ("task out"=w419:refnum<k21>, "error out"=w418:errorcluster)  [unwired: 12 in]
      n125 = Tick Count (ms)() -> (millisecond timer value=w432:u32)
      n126 = call-poly <vilib>:"DAQmx Write.vi"("task/channels in"=w396, "data"=TRUE, "error in"=w400) -> ("task out"=w399:refnum<k21>, "error out"=w398:errorcluster)  [unwired: 10 in, 1 out]
      n127 = call <vilib>:"DAQmx Start Task.vi"("task/channels in"=w425, "error in"=w424) -> ("task out"=w427:refnum<k21>, "error out"=w426:errorcluster)  [unwired: 12 in]
    }
  }
  n128 = To Long Integer(number=w231) -> (32bit integer=w230:i32)
  n129 = while {
    tunnel: [w487] -> w88
    tunnel: w306 -> [w487]
    tunnel: [w486] -> w87
    tunnel: w305 -> [w486]
    tunnel: w304 -> [w485]
    tunnel: w303 -> [w446]
    tunnel: w100 -> [w482]
    tunnel: [w482] -> w92
    tunnel: [w481] -> w91
    tunnel: w99 -> [w481]
    tunnel: [w480] -> w90
    tunnel: [w479] -> w89
    tunnel: w210 -> [w478]
    tunnel: w209 -> [w477]
    tunnel: w11 -> [w476]
    tunnel: w208 -> [w453]
    tunnel: w205 -> [w475]
    tunnel: w203 -> [w451]
    tunnel: w201 -> [w452]
    tunnel: w108 -> [w474]
    tunnel: w107 -> [w473]
    tunnel: [w462] -> w94
    tunnel: [w463] -> w95
    tunnel: w104 -> [w461]
    tunnel: w102 -> [w457]
    tunnel: [w457] -> w93
    tunnel: w11 -> [w454]
    tunnel: w11 -> [_]
    stop <- w484 stop-if-true
    # "Record from PCO"
    # "Write T/F \nto Solenoid\nArray"
    # "Track Time elapsed during trial"
    # "Record PCO"
    n130 = Tick Count (ms)() -> (millisecond timer value=w488:u32)
    n131 = call-dynamic "isRecording.vi"("Camera in"=w474, "error in (no error)"=w473) -> ("Camera out"=w472:refnum<class "Camera.lvclass">, "recording"=→"PCO Recording":bool, "error out"=w471:errorcluster)  [unwired: 11 in]
    n132 = Subtract(x=w488, y=w485) -> (x-y=w444:u32)
    n133 = call-dynamic "getRecordedImageCount.vi"("Camera in"=w472, "error in (no error)"=w471) -> ("Camera out"=w465:refnum<class "Camera.lvclass">, "recorded_image_count"=w449:u32, "error out"=w464:errorcluster)  [unwired: 11 in]
    "Recorded Images" <- w449
    n134 = Greater?(x=w449, y=w454) -> (0:w450:bool)
    n135 = case shown="True" w450 {
      tunnel: w453 -> [_ w505]
      tunnel: w475 -> [_ w495]
      tunnel: w476 -> [_ w500]
      tunnel: w452 -> [_ w502]
      tunnel: w451 -> [_ w501]
      tunnel: w449 -> [_ w496]
      tunnel: [w489 w497] -> w438
      frame False {
        w491 = FALSE
        n136 = Build Array(w491, FALSE, w491) -> (w489:bool[])
      }
      frame True {
        # "Track ISI"
        # "Track Solenoid\nOrder"
        # "Puffs"
        n137 = Subtract(x=w496, y=w500) -> (x-y=w499:dbl)
        n138 = Quotient & Remainder(x=w499, y=w505) -> (x-y*floor(x/y)=w506:dbl, floor(x/y)=w503:dbl)
        n139 = Quotient & Remainder(x=w503, y=w502) -> (x-y*floor(x/y)=w504:dbl)  [unwired: 1 out]
        n140 = Index Array(array=w501, index=w504) -> (element=w493:dbl)
        n141 = case shown="2" w493 {
          tunnel: [w507 w510 w513] -> w492
          frame 0, Default {
            w509 = TRUE
            n142 = Build Array(w509, FALSE, w509) -> (w507:bool[])
          }
          frame 1 {
            w512 = FALSE
            n143 = Build Array(w512, TRUE, w512) -> (w510:bool[])
          }
          frame 2 {
            w515 = FALSE
            n144 = Build Array(w515, FALSE, w515) -> (w513:bool[])
          }
        }
        n145 = In Range and Coerce(upper limit=w495, x=w506, lower limit=0.0) -> (In Range?=w498:bool)  [unwired: 1 out]
        n146 = And(x=w498, y=w492) -> (x .and. y?=w497:bool[])
      }
    }
    "Solenoids" <- w438
    n147 = Greater Or Equal?(x=w449, y=w461) -> (x >= y?=w460:bool)
    n148 = Divide(x=w444, y=1000.0) -> (x/y=w440:dbl)
    "Time Elapsed (s)" <- w440
    n149 = local read "Image"() -> (w448:T3)
    n150 = Divide(x=w449, y=w440) -> (x/y=→"PCO Frame Rate":dbl)
    n151 = call-dynamic "image.vi"("Camera in"=w465, "data_format"=T14."Mono16", "image_index"=u32 4294967295 ("dwImgIdx"), "error in (no error)"=w464) -> ("Camera out"=w462:refnum<class "Camera.lvclass">, "raw_image (U16)"=w466:u16[][], "error out"=w463:errorcluster)  [unwired: 4 in, 5 out]
    n152 = Divide(x=w446, y=60.0) -> (x/y=w442:dbl)
    n153 = local write "Stop"("Stop") -> ()
    n154 = Divide(x=w440, y=60.0) -> (x/y=w439:dbl)
    n155 = call "IMAQ ArrayToImage"("Image Pixels (U16)"=w466, "Image"=w448) -> ("error out"=w468:errorcluster, "Image Out"=w447:T3)  [unwired: 8 in]
    n156 = Bundle(w442, w439) -> (→"Trial Time Elapsed (Min)":cluster{dbl, dbl})  [unwired: 1 in]
    n157 = local write "Image"(w447) -> ()
    n158 = Unbundle By Name(w468) -> ("status"=w459:bool)
    n159 = Unbundle By Name(w463) -> ("status"=w458:bool)
    n160 = Compound Arithmetic op=OR("Stop", w460, w459, w458) -> (w484:bool)
    "CBV Camera" <- w484
    n161 = call-poly <vilib>:"DAQmx Write.vi"("task/channels in"=w478, "data"=w438, "error in"=w477) -> ("task out"=w480:refnum<k21>, "error out"=w479:errorcluster)  [unwired: 10 in, 1 out]
  }
  n162 = while {
    tunnel: w319 -> [w528]
    tunnel: w313 -> [w521]
    tunnel: w311 -> [w527]
    tunnel: w309 -> [w526]
    tunnel: w307 -> [w522]
    tunnel: [w525] -> w84
    tunnel: [w524] -> w86
    tunnel: [w523] -> w85
    i -> [w520]
    stop <- w529 stop-if-true
    # "Record Webcam"
    n163 = Quotient & Remainder(x=w520, y=2) -> (x-y*floor(x/y)=w518:i32)  [unwired: 1 out]
    n164 = Less Or Equal?(x=w518, y=0) -> (x <= y?=w516:bool)
    n165 = case shown="True" w516 {
      tunnel: w528 -> [_ w543]
      tunnel: w527 -> [w532 w542]
      tunnel: w526 -> [w531 w538]
      tunnel: [w532 w537] -> w525
      tunnel: [w531 w535] -> w524
      tunnel: [w530 w533] -> w523
      tunnel: w522 -> [w530 w533]
      tunnel: w521 -> [_ w541]
      tunnel: w520 -> [_ w540]
      frame False {
      }
      frame True {
        n166 = Tick Count (ms)() -> (millisecond timer value=w546:u32)
        n167 = Subtract(x=w546, y=w543) -> (x-y=w547:u32)
        n168 = Divide(x=w547, y=u32 1000) -> (x/y=w539:dbl)
        n169 = call "WebCam Grab_FLIR_trig.vi"("Session In"=w542, "Image In"=w541, "Buffer Number In"=w540, "Trial Time"=w539, "AVI Refnum"=w533, "error in"=w538) -> ("Session Out"=w537:T5, "WebCam Img Out"=→"WebCam":T3, "Buffer Number Out"=w534:u32, "error out"=w535:errorcluster)  [unwired: 10 in]
        n170 = call <vilib>:"Calculate Frames per Second.vi"("Update Interval (ms)"=u32 5000, "Buffer Number"=w534) -> ("Processed Frames/s"=→"Actual WebCam Frame Rate":dbl)  [unwired: 7 in, 2 out]
      }
    }
    n171 = local read "CBV Camera"() -> (w529:bool)
  }
  n172 = while {
    tunnel: w175 -> [w568]
    tunnel: [w569] -> w80
    tunnel: w174 -> [w569]
    tunnel: [w568] -> w81
    tunnel: [w551] -> w82
    tunnel: [w553] -> w75
    tunnel: [w567] -> w74
    tunnel: w172 -> [w566]
    tunnel: w170 -> [w565]
    tunnel: w161 -> [w564]
    tunnel: w158 -> [w563]
    shift-right: [w562] -> w6
    shift-left: u32 0 ("Buffer Number Out") -> [w561]
    shift-right: [w560] -> w3
    shift-left: u32 0 ("New Lost") -> [w559]
    shift-right: [w558] -> w5
    shift-left: u32[] [] ("NewBuffNum") -> [w557]
    shift-right: [w556] -> w4
    shift-left: u32[] [] ("NewNumLost") -> [w555]
    stop <- w554 stop-if-true
    # "Track Dropped Frames"
    # "Record auxiliary camera (whiskers/pupil depending on setup)"
    n173 = call <vilib>:"IMAQdx Get Image.vi"("Buffer Number Mode (Next)"=IMAQdx_Buffer_Number_Mode."Next", "error in"=w565, "Image In"=w564, "Session In"=w566) -> ("error out"=w576:errorcluster, "Buffer Number Out"=w562:u32, "Image Out"=w549:T3, "Session Out"=w551:T5)  [unwired: 4 in]
    "Last Whisk\nBuffer" <- w562
    "Pupil" <- w549
    n174 = call "Track Dropped Frames_atw1.vi"("NumLost"=w555, "BuffNum"=w557, "Curr Buffer"=w562, "Prev Lost"=w559, "Prev Buffer"=w561) -> ("New Lost"=w560:u32, "NewNumLost"=w556:u32[], "NewBuffNum"=w558:u32[])  [unwired: 4 in]
    n175 = local read "CBV Camera"() -> (w550:bool)
    n176 = call "IMAQ ImageToArray"("error in (no error)"=w576, "Image"=w549) -> ("error out"=w575:errorcluster, "Image Pixels (U8)"=w574:u8[][])  [unwired: 2 in, 3 out]
    n177 = call <vilib>:"Calculate Frames per Second.vi"("Update Interval (ms)"=u32 2000, "Buffer Number"=w562) -> ("Processed Frames/s"=→"Actual WhiskCam\nFrame Rate":dbl)  [unwired: 7 in, 2 out]
    n178 = Write to Binary File(file (use dialog)=w563, data=w574, error in=w575, 5:FALSE ("prepend array or string size? (T)"), 9:T15."little-endian" ("byte order (0:big-endian, network order)")) -> (refnum out=w567:refnum<file>, error out=w553:errorcluster)  [unwired: 1 in, 1 out]
    n179 = Unbundle By Name(w553) -> ("status"=w552:bool)
    n180 = Or(x=w552, y=w550) -> (x .or. y?=w554:bool)
  }
  "Buffer Number Out" <- w6
  "NewBuffNum" <- w5
  "NewNumLost" <- w4
  "New Lost" <- w3
  n181 = while {
    tunnel: w290 -> [w597]
    tunnel: w289 -> [w596]
    tunnel: w287 -> [w595]
    tunnel: [w594] -> w76
    tunnel: [w578] -> w77
    tunnel: [w593] -> w83
    shift-right: [w585] -> _
    shift-left: 0 -> [w586]
    tunnel: w230 -> [w584]
    stop <- w580 stop-if-true
    # "Record Analog Data"
    n182 = call-poly <vilib>:"DAQmx Read.vi"("task/channels in"=w596, "error in"=w597) -> ("task out"=w593:refnum<k21>, "data"=w591:waveform(dbl)[], "error out"=w583:errorcluster)  [unwired: 11 in]
    n183 = Index Array(array=w591, index=0) -> (element=w589:waveform(dbl))
    n184 = Unbundle By Name(w589) -> ("Y"=w588:dbl[])
    n185 = Array Size(array=w588) -> (size(s)=w587:i32)
    n186 = local read "Stop"() -> (w581:bool)
    n187 = local read "CBV Camera"() -> (w579:bool)
    n188 = Add(x=w587, y=w586) -> (x+y=w585:i32)
    "Analog acquisition length" <- w585
    n189 = Greater Or Equal?(x=w585, y=w584) -> (x >= y?=w582:bool)
    n190 = TDMS Write(0:w595, 5:"Analog Data" ("group name in (Untitled)"), 9:w591, 11:w583) -> (4:w594:refnum<k34>, 15:w578:errorcluster)  [unwired: 2 in, 2 out]
    n191 = Compound Arithmetic op=OR(w578, w582, w581, w579) -> (w580:bool)
    "Analog Data" <- w580
  }
  n192 = while {
    shift-right: [w625] -> _
    shift-left: enum16{"Close all devices", "Move files"}."Close all devices" ("Enum") -> [w626]
    tunnel: w94 -> [w623]
    tunnel: w93 -> [w622]
    tunnel: w92 -> [w621]
    tunnel: w91 -> [w620]
    tunnel: w90 -> [w619]
    tunnel: w89 -> [w618]
    tunnel: w88 -> [w617]
    tunnel: w87 -> [w616]
    tunnel: w85 -> [w614]
    tunnel: w84 -> [w613]
    tunnel: w83 -> [w612]
    tunnel: w82 -> [w609]
    tunnel: w81 -> [w608]
    tunnel: w80 -> [w607]
    tunnel: w79 -> [w606]
    shift-right: [w599] -> w71
    shift-left: w86 -> [w615]
    tunnel: "Target Path" -> [w605]
    tunnel: w76 -> [w604]
    shift-right: [w600] -> w72
    shift-left: w77 -> [w611]
    tunnel: w74 -> [w603]
    shift-right: [w601] -> w73
    shift-left: w75 -> [w610]
    shift-right: [w598] -> w70
    shift-left: w95 -> [w624]
    stop <- w602 stop-if-true
    # "Close, save & exit"
    n193 = case shown="\"Close all devices\", Default" w626 {
      tunnel: [enum16{"Close all devices", "Move files"}."Move files" ("Enum") enum16{"Close all devices", "Move files"}."Close all devices" ("Enum")] -> w625
      tunnel: w624 -> [w660 w663]
      tunnel: w623 -> [w659 _]
      tunnel: w622 -> [_ w685]
      tunnel: w621 -> [w654 _]
      tunnel: w620 -> [w652 _]
      tunnel: w619 -> [w630 _]
      tunnel: w618 -> [w628 _]
      tunnel: w617 -> [w649 _]
      tunnel: w616 -> [w648 _]
      tunnel: w615 -> [w646 w683]
      tunnel: w614 -> [w647 _]
      tunnel: w613 -> [w645 _]
      tunnel: w612 -> [w644 _]
      tunnel: w611 -> [w643 w675]
      tunnel: w610 -> [w641 w670]
      tunnel: w609 -> [w640 _]
      tunnel: w608 -> [w639 _]
      tunnel: w607 -> [w638 _]
      tunnel: w606 -> [_ w684]
      tunnel: w605 -> [_ w671]
      tunnel: w604 -> [_ w662]
      tunnel: w603 -> [_ w672]
      tunnel: [FALSE TRUE] -> w602
      tunnel: [w633 w667] -> w601
      tunnel: [w634 w666] -> w600
      tunnel: [w635 w665] -> w599
      tunnel: [w632 w664] -> w598
      frame "Close all devices", Default {
        # "occasionally the trial\nends with the puffer left on\nunless we explicitly write falses\nto all stim lines"
        # "next loop: handle files"
        # "Stop PCO recording and release resources\n\nNOTE: IF THIS IS NOT RUN AT \nTHE END OF EVERY TRIAL, THE\nCAMERA WILL BE DEADLOCKED\nIN A RECORDING SESSION AND \nYOU WILL HAVE TO RESTART THE CAMERA\nAND/OR COMPUTER TO RESET IT\n\n(this wastes a lot of time)"
        # "Stop & clear start trigger"
        # "Stop & clear sensory stim output"
        # "Stop counter task"
        # "Close video object\n& release resources"
        # "Close webcam AVI"
        # "Close video object & release resources"
        # "Stop camera acquisition"
        # "Stop & clear analog acquisition task"
        # "-1 will release the buffer."
        n194 = call-dynamic "close.vi"("error in (no error)"=w660, "Camera in"=w659) -> ("error out"=w632:errorcluster)  [unwired: 9 in]
        n195 = call <vilib>:"DAQmx Stop Task.vi"("task/channels in"=w649, "error in"=w648) -> ()  [unwired: 12 in, 2 out]
        n196 = call <vilib>:"IMAQdx Close Camera.vi"("error in"=w641, "Session In"=w640) -> ("error out"=w633:errorcluster)  [unwired: 9 in]
        n197 = call-poly <vilib>:"DAQmx Write.vi"("task/channels in"=w654, "data"=FALSE, "error in"=w652) -> ("task out"=w655:refnum<k21>, "error out"=w657:errorcluster)  [unwired: 10 in, 1 out]
        n198 = call <vilib>:"DAQmx Stop Task.vi"("task/channels in"=w639, "error in"=w638) -> ()  [unwired: 12 in, 2 out]
        n199 = call <vilib>:"DAQmx Stop Task.vi"("task/channels in"=w644, "error in"=w643) -> ("task out"=w642:refnum<k21>, "error out"=w637:errorcluster)  [unwired: 12 in]
        n200 = call "IMAQ AVI2 Close"("error in (no error)"=w646, "AVI Refnum"=w647) -> ("error out"=w635:errorcluster)  [unwired: 9 in]
        n201 = call <vilib>:"IMAQdx Close Camera.vi"("error in"=w646, "Session In"=w645) -> ()  [unwired: 9 in, 1 out]
        n202 = call-poly <vilib>:"DAQmx Write.vi"("task/channels in"=w630, "data"=bool[] [FALSE, FALSE, FALSE], "error in"=w628) -> ("task out"=w629:refnum<k21>, "error out"=w627:errorcluster)  [unwired: 10 in, 1 out]
        n203 = call <vilib>:"DAQmx Stop Task.vi"("task/channels in"=w655, "error in"=w657) -> ("task out"=w656:refnum<k21>, "error out"=w658:errorcluster)  [unwired: 12 in]
        n204 = call <vilib>:"DAQmx Clear Task.vi"("task in"=w642, "error in"=w637) -> ("error out"=w634:errorcluster)  [unwired: 13 in]
        n205 = call <vilib>:"DAQmx Clear Task.vi"("task in"=w656, "error in"=w658) -> ()  [unwired: 13 in, 1 out]
        n206 = call <vilib>:"DAQmx Stop Task.vi"("task/channels in"=w629, "error in"=w627) -> ("task out"=w651:refnum<k21>, "error out"=w650:errorcluster)  [unwired: 12 in]
        n207 = call <vilib>:"DAQmx Clear Task.vi"("task in"=w651, "error in"=w650) -> ()  [unwired: 13 in, 1 out]
      }
      frame "Move files" {
        # "(shouldn't run)"
        n208 = Path To String(path=w685) -> (string=w687:string)
        n209 = Close File(refnum=w672, error in=w670) -> (path=w673:path, error out=w674:errorcluster)
        n210 = Concatenate Strings(w687, "_Cam01.pcoraw" ("string")) -> (w688:string)
        n211 = TDMS Close(8:w675, 11:w662) -> (0:w677:errorcluster, 3:w679:path)
        n212 = String To Path(string=w688) -> (path=w689:path)
        n213 = Move(source path=w684, error in=w683, 10:w671) -> (error out=w665:errorcluster)  [unwired: 2 in, 2 out]
        n214 = TDMS Defragment(4:w677, 7:w679) -> (0:w682:errorcluster)
        n215 = Move(source path=w673, error in=w674, 10:w671) -> (error out=w667:errorcluster)  [unwired: 2 in, 2 out]
        n216 = Path To String(path=w679) -> (string=w678:string)
        n217 = Move(source path=w689, error in=w663, 10:w671) -> (error out=w664:errorcluster)  [unwired: 2 in, 2 out]
        n218 = Concatenate Strings(w678, "_index" ("string")) -> (w680:string)
        n219 = String To Path(string=w680) -> (path=w681:path)
        n220 = Move(source path=w679, error in=w682, 10:w671) -> (error out=w666:errorcluster)  [unwired: 2 in, 2 out]
        n221 = Move(source path=w681, error in=w682, 10:w671) -> ()  [unwired: 2 in, 3 out]
      }
    }
  }
  n222 = call <vilib>:"Simple Error Handler.vi"("error in (no error)"=w73) -> ()  [unwired: 1 in, 8 out]
  n223 = call <vilib>:"Simple Error Handler.vi"("error in (no error)"=w70) -> ()  [unwired: 1 in, 8 out]
  n224 = call <vilib>:"Simple Error Handler.vi"("error in (no error)"=w71) -> ()  [unwired: 1 in, 8 out]
  n225 = call <vilib>:"Simple Error Handler.vi"("error in (no error)"=w72) -> ()  [unwired: 1 in, 8 out]
